vi "Equip-Get AO Channels (String).vi"(0 "section":string="Connections", 2 "Path":path, 7 "Channel Names":string[](array[string]), 11 "error in (no error)":errorcluster) -> (8 "AO Channels":i32[](array[numeric]), 15 "error out":errorcluster)   [LabVIEW 2020]
uses:
  <vilib>/Utility/config.llb/Read Key (I32).vi
  <vilib>/Utility/config.llb/NI_LVConfig.lvlib
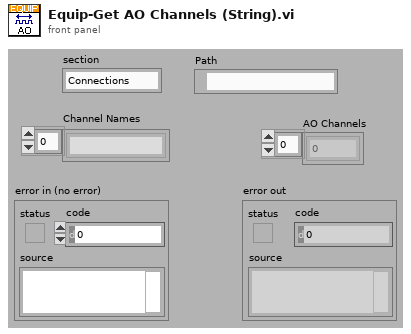
[diagram p1: front panel]
types:
  T1 = typedef "NI_LVConfig.lvlib/Config Data RefNum.ctl" = refnum<k1>
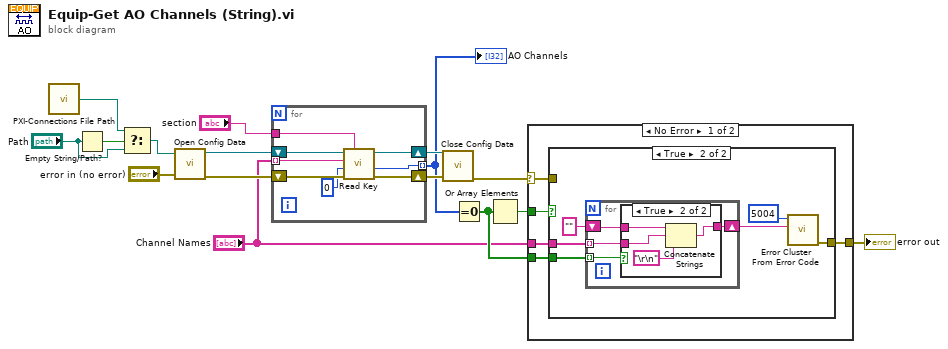
[diagram p0: block diagram]
diagram:
  n1 = call "PXI-Connections File Path.vi"() -> ("Path"=w3:path)  [unwired: 1 in]
  n2 = Empty String/Path?(string/path="Path") -> (empty?=w4:bool)
  n3 = Select(t=w3, s=w4, f="Path") -> (s? t:f=w1:path)
  n4 = call <vilib>:"Open Config Data.vi"("error in (no error)"="error in (no error)", "configuration file path"=w1) -> ("error out"=w6:errorcluster, "refnum"=w9:T1)  [unwired: 7 in, 1 out]
  n5 = for {
    tunnel: [w21] -> w13 mode=indexing
    shift-right: [w20] -> w15
    shift-left: w6 -> [w24]
    tunnel: "section" -> [w18]
    tunnel: "Channel Names" -> [w17] mode=indexing
    shift-right: [w19] -> w14
    shift-left: w9 -> [w23]
    n6 = call-poly <vilib>:"Read Key.vi"("section"=w18, "error in (no error)"=w24, "default value"=0, "key"=w17, "refnum"=w23) -> ("error out"=w20:errorcluster, "value"=w21:i32, "refnum out"=w19:T1)  [unwired: 3 in, 1 out]
  }
  "AO Channels" <- w13
  n7 = call <vilib>:"Close Config Data.vi"("error in (no error)"=w15, "refnum"=w14) -> ("error out"=w10:errorcluster)  [unwired: 8 in, 1 out]
  n8 = Equal To 0?(x=w13) -> (x = 0?=w7:bool[])
  n9 = Or Array Elements(Boolean array=w7) -> (logical OR=w12:bool)
  n10 = case shown="No Error" w10 {
    selector: w10 -> [w27 w46]
    tunnel: w12 -> [w29 _]
    tunnel: [w28 w46] -> w11
    tunnel: "Channel Names" -> [w26 _]
    tunnel: w7 -> [w25 _]
    frame No Error {
      n11 = case shown="True" w29 {
        tunnel: w27 -> [w30 _]
        tunnel: [w30 w35] -> w28
        tunnel: w26 -> [_ w36]
        tunnel: w25 -> [_ w32]
        frame False {
        }
        frame True {
          n12 = for {
            tunnel: w36 -> [w39] mode=indexing
            shift-right: [w40] -> w34
            shift-left: "" -> [w38]
            tunnel: w32 -> [w37] mode=indexing
            n13 = case shown="True" w37 {
              tunnel: [w41 w45] -> w40
              tunnel: w39 -> [_ w44]
              tunnel: w38 -> [w41 w43]
              frame False {
              }
              frame True {
                n14 = Concatenate Strings(w43, w44, "\r\n") -> (w45:string)
              }
            }
          }
          n15 = call <vilib>:"Error Cluster From Error Code.vi"("error message (\"\")"=w34, "error code (0)"=5004) -> ("error out"=w35:errorcluster)  [unwired: 7 in]
        }
      }
    }
    frame Error {
    }
  }
  "error out" <- w11
